vi "Get Connected.vi"(8 "error in (no error)":errorcluster, 11 "VISA Client in":refnum<class "Serial Client.lvclass">) -> (0 "error out":errorcluster, 2 "Connected":bool, 3 "VISA Client out":refnum<class "Serial Client.lvclass">)   [LabVIEW 2020, in "Stream-Serial.lvlib" / "Serial Client.lvclass"]
uses:
  Serial Client.lvclass
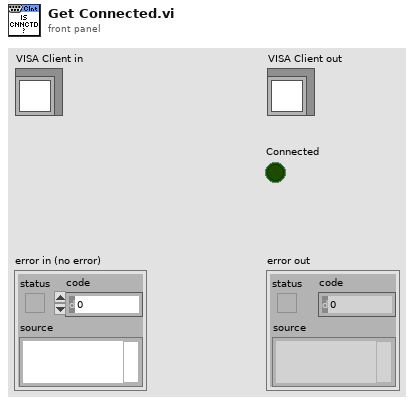
[diagram p1: front panel]
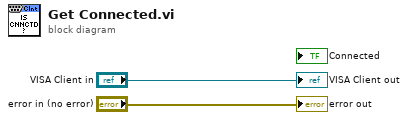
[diagram p0: block diagram]
diagram:
  "error out" <- "error in (no error)"
  "VISA Client out" <- "VISA Client in"
